vi "MinPred.vi"(8 "error in (no error)":errorcluster, 10 "node ref in":refnum<data-value>, 11 "RVCLibrary_Bug in":refnum<class "RVCLibrary_Bug2.lvclass">) -> (0 "error out":errorcluster, 1 "cost of node to min pred":dbl, 2 "min node ref":refnum<data-value>, 3 "RVCLibrary_Bug out":refnum<class "RVCLibrary_Bug2.lvclass">)   [LabVIEW 2013, in "RVCLibrary_Bug2.lvclass"]
uses:
  RVCLibrary_Bug2.lvclass
  <vilib>/robotics/Navigation/shared/MapNode/AbstractDstarNode/NI_Robotics_AbstractDstarNode.lvclass
  <vilib>/robotics/Navigation/shared/WorldMap/AbstractWorldMap/NI_Robotics_AbstractWorldMap.lvclass
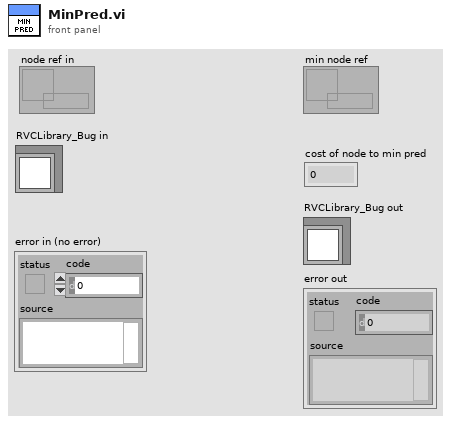
[diagram p1: front panel]
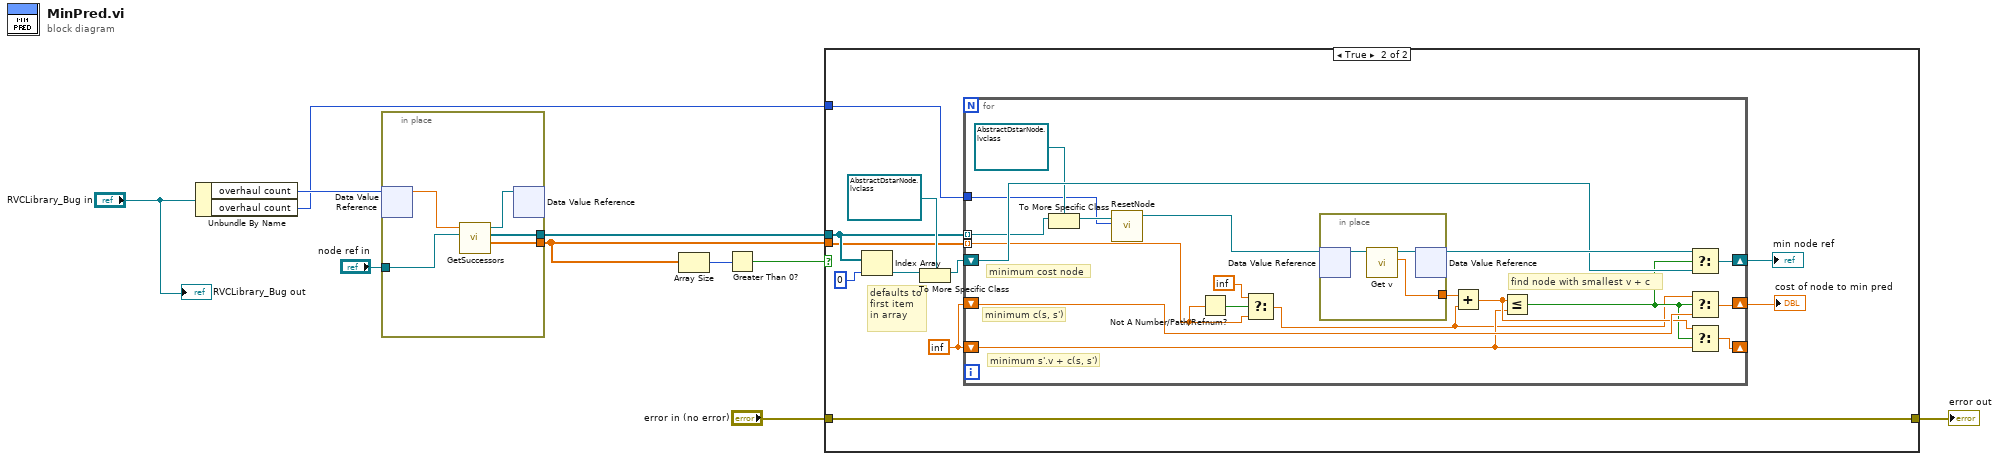
[diagram p0: block diagram]
diagram:
  n1 = Unbundle By Name("RVCLibrary_Bug in") -> ("overhaul count"=w9:i32, "overhaul count"=w4:i32)
  n2 = in-place {
    in-place-border: "node ref in" -> [w14]
    in-place-border: [w12] -> w7
    in-place-border: [w11] -> w5
    n3 = in-place-dvr #1(w9) -> (w15:dbl)  [unwired: 1 out]
    n4 = call-dynamic "GetSuccessors.vi"("AbstractMapNode Ref"=w14, "WorldMap in"=w15) -> ("EdgeCost"=w11:dbl[], "Successors"=w12:refnum<data-value>[], "WorldMap out"=w13:refnum<class "NI_Robotics_AbstractWorldMap.lvclass">)  [unwired: 6 in, 1 out]
    n5 = in-place-dvr #1(w13) -> ()  [unwired: 2 out]
  }
  n6 = Array Size(array=w5) -> (size(s)=w8:i32)
  n7 = Greater Than 0?(x=w8) -> (x > 0?=w6:bool)
  n8 = case shown="True" w6 {
    tunnel: w7 -> [_ w20]
    tunnel: w5 -> [_ w19]
    tunnel: w4 -> [_ w18]
    tunnel: "error in (no error)" -> [w16 w17]
    tunnel: [w16 w17] -> w2
    frame False {
    }
    frame True {
      w25 = inf
      # "defaults to\nfirst item\nin array"
      n9 = Index Array(array=w20, index=0) -> (element=w23:refnum<data-value>)
      n10 = To More Specific Class(target class=refnum<data-value> refnum ("data value reference"), reference=w23) -> (specific class reference=w22:refnum<data-value>)  [unwired: 1 in, 1 out]
      n11 = for {
        tunnel: w20 -> [w30] mode=indexing
        tunnel: w19 -> [w33] mode=indexing
        shift-right: [w45] -> _
        shift-left: w25 -> [w38]
        shift-right: [w44] -> w27
        shift-left: w22 -> [w42]
        shift-right: [w40] -> w26
        shift-left: w25 -> [w41]
        tunnel: w18 -> [w29]
        # "minimum s'.v + c(s, s')"
        # "minimum c(s, s')"
        # "minimum cost node"
        # "find node with smallest v + c"
        n12 = To More Specific Class(target class=refnum<data-value> refnum ("node reference in"), reference=w30) -> (specific class reference=w31:refnum<data-value>)  [unwired: 1 in, 1 out]
        n13 = call "ResetNode.vi"("overhaul count"=w29, "node reference in"=w31) -> ("node reference out"=w28:refnum<data-value>)  [unwired: 9 in]
        n14 = Not A Number/Path/Refnum?(number/path/refnum=w33) -> (NaN/Path/Refnum?=w34:bool)
        n15 = Select(t=inf, s=w34, f=w33) -> (s? t:f=w36:dbl)
        n16 = in-place {
          in-place-border: [w47] -> w46
          n17 = in-place-dvr #2(w28) -> (w49:refnum<class "NI_Robotics_AbstractDstarNode.lvclass">)  [unwired: 1 out]
          n18 = call <vilib>:"Get v.vi"("AbstractDstarNode in"=w49) -> ("v"=w47:dbl, "AbstractDstarNode out"=w48:refnum<class "NI_Robotics_AbstractDstarNode.lvclass">)  [unwired: 9 in]
          n19 = in-place-dvr #2(w48) -> (w43:refnum<data-value>)  [unwired: 1 out]
        }
        n20 = Add(x=w46, y=w36) -> (x+y=w39:dbl)
        n21 = Less Or Equal?(x=w39, y=w38) -> (x <= y?=w37:bool)
        n22 = Select(t=w43, s=w37, f=w42) -> (s? t:f=w44:refnum<data-value>)
        n23 = Select(t=w36, s=w37, f=w41) -> (s? t:f=w40:dbl)
        n24 = Select(t=w39, s=w37, f=w38) -> (s? t:f=w45:dbl)
      }
      "min node ref" <- w27
      "cost of node to min pred" <- w26
    }
  }
  "error out" <- w2
  "RVCLibrary_Bug out" <- "RVCLibrary_Bug in"
